vi "Initialize Stop Event.vi"   [LabVIEW 2013]
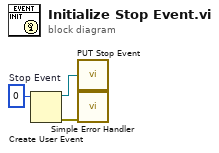
[diagram p0: block diagram]
diagram:
  w3 = 0  # Stop Event
  n1 = Create User Event(user event datatype=w3) -> (user event=w2:refnum<user-event>, error out=w1:errorcluster)  [unwired: 1 in]
  n2 = call "PUT Stop Event.vi"("Stop Event"=w2) -> ()
  n3 = call <vilib>:"Simple Error Handler.vi"("error in (no error)"=w1) -> ()  [unwired: 4 in, 5 out]
